vi "RD Calibration Write.vi"(8 "error in (no error)":errorcluster caption="错误输入（无错误）", 10 "CalArray":i32[](array[numeric])=[0, 0, 0, 0, 0, 0, 0, 0, 0, 0, 0, 0, 0, 0, 0, 0, 0], 11 "handle":u64) -> (0 "error out":errorcluster caption="错误输出", 1 "function return":i32, 2 "CalArray out":i32[](array[numeric]), 3 "handle out":u64)   [LabVIEW 2018, in "InstrumentsPlayground.lvlib"]
doc: "CLIFFAPI int CliffCalibrationWrite(FT_HANDLE handle,int *CalArray);"
uses:
  InstrumentsPlayground.lvlib
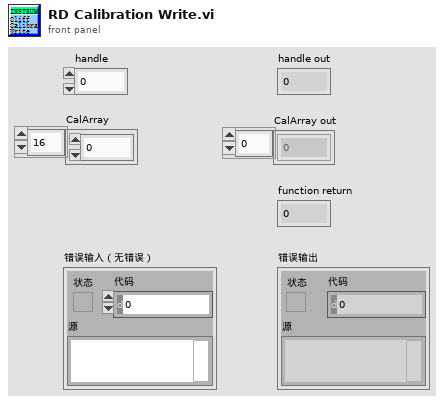
[diagram p1: front panel]
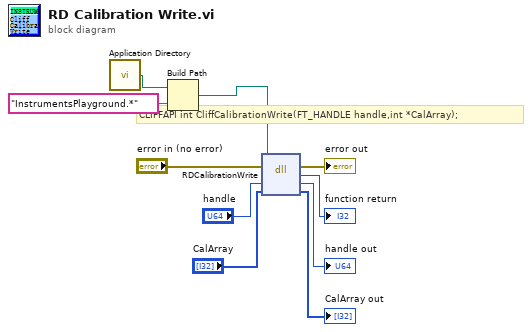
[diagram p0: block diagram]
diagram:
  # "CLIFFAPI int CliffCalibrationWrite(FT_HANDLE handle,int *CalArray);"
  n1 = call <vilib>:"Application Directory.vi"() -> ("Application Directory"=w2:path)
  n2 = Build Path(base path=w2, name or relative path="InstrumentsPlayground.*" ("名称或相对路径")) -> (appended path=w1:path)
  n3 = dll-call lib="E:/Work/YZCourse_Xtext/Cliff/API/IPLabView lib/InstrumentsPlayground.*" fn="RDCalibrationWrite"(path in=w1, error in="error in (no error)", "handle"="handle", "CalArray"="CalArray") -> (error out=→"error out":errorcluster, "返回类型"=→"function return":i32, "handle"=→"handle out":u32, "CalArray"=→"CalArray out":i32[])  [unwired: 1 in, 1 out]
